vi "Vel Override.vi"(4 "Jerk Multiplier":dbl=100.0 format="%#_13g", 5 "VEL ADJ":dbl, 6 "Acc Multiplier":dbl=10.0 format="%#_13g", 8 "error in (no error)":errorcluster, 9 "CMD In":T1, 10 "Motion Parameters (Default)":T2={"timeout"=-1.0, "acceleration"=10000.0, "deceleration"=10000.0, "accel. jerk"=100000.0, "decel. jerk"=100000.0, "blend mode"=10551334, "blend delay"=-1.0, "smoothing"=0.5, "last blend"=FALSE} {"blend mode" items=["At Profile Complete"=10551335, "At Deceleration"=10551334, "After Delay"=10551336]}) -> (0 "error out":errorcluster, 1 "CMD Out":T1, 2 "output cluster":T2={"timeout"=-1.0, "acceleration"=10000.0, "deceleration"=10000.0, "accel. jerk"=100000.0, "decel. jerk"=100000.0, "blend mode"=10551334, "blend delay"=-1.0, "smoothing"=0.5, "last blend"=FALSE} {"blend mode" items=["At Profile Complete"=10551335, "At Deceleration"=10551334, "After Delay"=10551336]})   [LabVIEW 2014]
uses:
  GCode Parser/GCode Command Cluster.ctl
  Typedefs/Motion Parameters.ctl
  <vilib>/Motion/Express/_s/nimc.fb.straightLineMove.blendMode.ctl
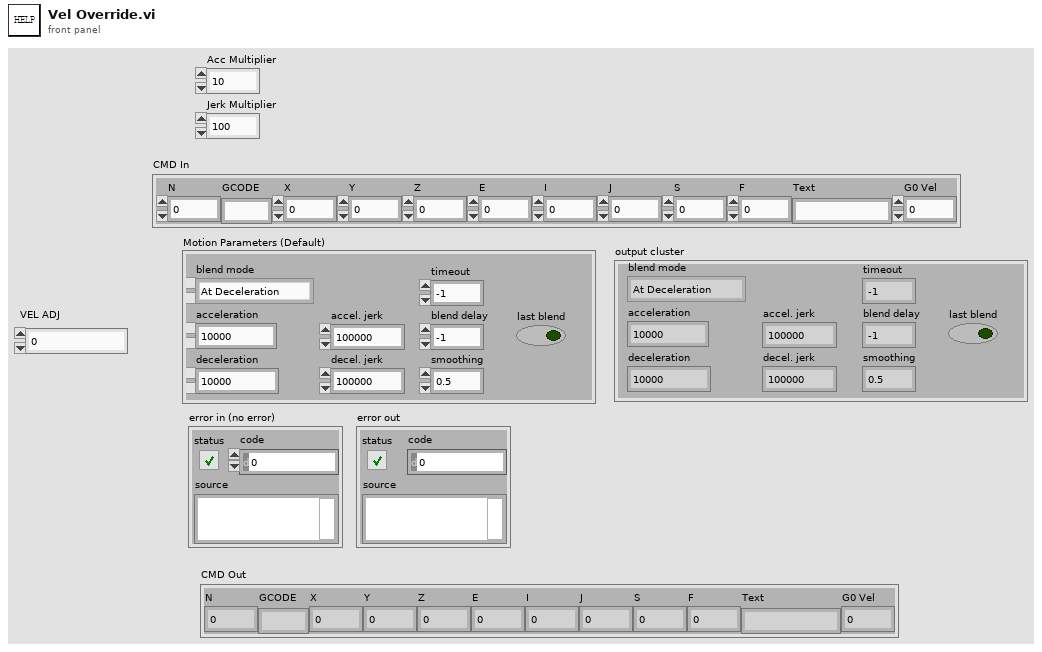
[diagram p1: front panel]
types:
  T1 = typedef "GCode Command Cluster.ctl" = cluster{"N":dbl, "GCODE":string, "X":dbl, "Y":dbl, "Z":dbl, "E":dbl, "I":dbl, "J":dbl, "S":dbl, "F":dbl, "Text":string, "G0 Vel":dbl}
  T2 = typedef "Motion Parameters.ctl" = cluster{"timeout":dbl, "acceleration":dbl, "deceleration":dbl, "accel. jerk":dbl, "decel. jerk":dbl, "blend mode":T3, "blend delay":dbl, "smoothing":dbl, "last blend":bool}
  T3 = typedef "nimc.fb.straightLineMove.blendMode.ctl" = i32
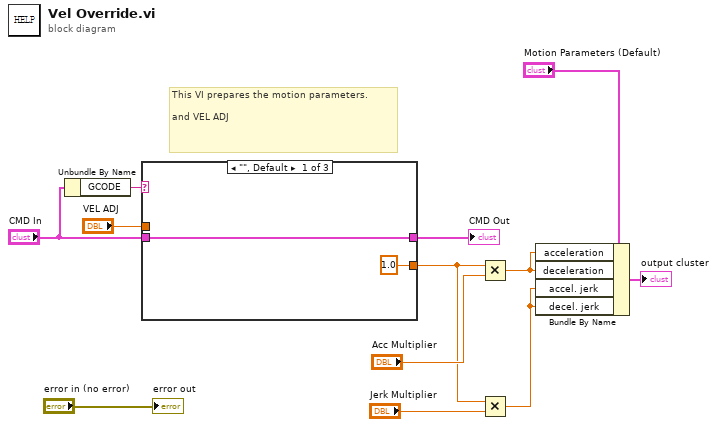
[diagram p0: block diagram]
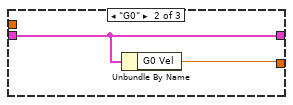
[diagram p2: hidden frame]
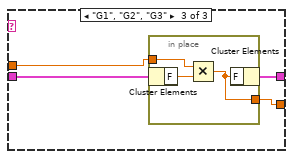
[diagram p3: hidden frame]
diagram:
  # "This VI prepares the motion parameters.\n\nand VEL ADJ"
  n1 = Unbundle By Name("CMD In") -> ("GCODE"=w1:string)
  n2 = case shown="\"\", Default" w1 {
    tunnel: "CMD In" -> [w14 w16 w17]
    tunnel: "VEL ADJ" -> [_ _ w20]
    tunnel: [w14 w16 w19] -> w4
    tunnel: [1.0 ("G0 Velocity") w15 w18] -> w3
    frame "", Default {
    }
    frame "G0" {
      n3 = Unbundle By Name(w16) -> ("G0 Vel"=w15:dbl)
    }
    frame "G1", "G2", "G3" {
      n4 = in-place {
        in-place-border: w20 -> [w22]
        in-place-border: [w21] -> w18
        n5 = in-place-cluster #1(w17) -> ("F"=w23:dbl)
        n6 = Multiply(x=w22, y=w23) -> (x*y=w21:dbl)
        n7 = in-place-cluster #1("F"=w21) -> (w19:T1)
      }
    }
  }
  "CMD Out" <- w4
  n8 = Multiply(x=w3, y="Acc Multiplier") -> (x*y=w9:dbl)
  n9 = Multiply(x=w3, y="Jerk Multiplier") -> (x*y=w8:dbl)
  n10 = Bundle By Name(cluster="Motion Parameters (Default)", "acceleration"=w9, "deceleration"=w9, "accel. jerk"=w8, "decel. jerk"=w8) -> (→"output cluster":T2)
  "error out" <- "error in (no error)"
